vi "CTRE_PID.vi"(9 "Sensor Derivative":dbl, 10 "Servo Params":T1, 11 "Error":dbl) -> (2 "At Target":bool, 3 "Out":dbl)   [LabVIEW 2016]
uses:
  <vilib>/Rock Robotics/WPI/ThirdParty/CanMotor/CTRLib-LV-TalonSRX/Framework/ServoParams.ctl
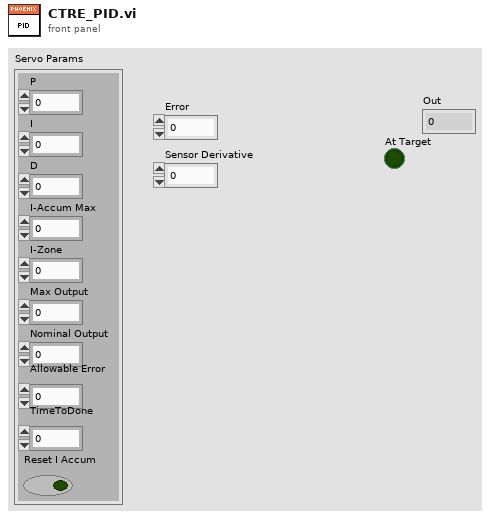
[diagram p1: front panel]
types:
  T1 = typedef "ServoParams.ctl" = cluster{"P":dbl, "I":dbl, "D":dbl, "I-Accum Max":dbl, "I-Zone":dbl, "Max Output":dbl, "Nominal Output":dbl, "Allowable Error":dbl, "TimeToDone":dbl, "Reset I Accum":bool}
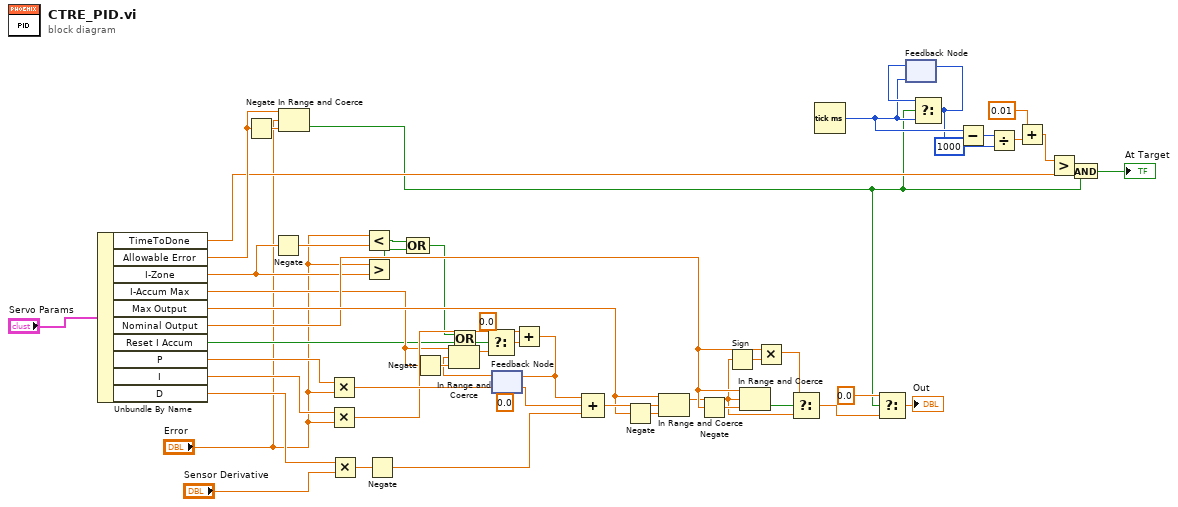
[diagram p0: block diagram]
diagram:
  n1 = Unbundle By Name("Servo Params") -> ("TimeToDone"=w10:dbl, "Allowable Error"=w17:dbl, "I-Zone"=w23:dbl, "I-Accum Max"=w29:dbl, "Max Output"=w38:dbl, "Nominal Output"=w35:dbl, "Reset I Accum"=w26:bool, "P"=w48:dbl, "I"=w47:dbl, "D"=w43:dbl)
  n2 = Negate(x=w17) -> (-x=w18:dbl)
  n3 = Negate(x=w23) -> (-x=w22:dbl)
  n4 = In Range and Coerce(upper limit=w17, x="Error", lower limit=w18) -> (In Range?=w6:bool)  [unwired: 1 out]
  n5 = Multiply(x=w48, y="Error") -> (x*y=w46:dbl)
  n6 = Multiply(x=w47, y="Error") -> (x*y=w45:dbl)
  n7 = Multiply(x=w43, y="Sensor Derivative") -> (x*y=w25:dbl)
  n8 = Less?(x="Error", y=w22) -> (x < y?=w20:bool)
  n9 = Greater?(x="Error", y=w23) -> (0:w21:bool)
  n10 = Negate(x=w25) -> (-x=w24:dbl)
  n11 = Compound Arithmetic op=OR(w20, w21) -> (w19:bool)
  n12 = Negate(x=w29) -> (-x=w31:dbl)
  n13 = Or(x=w19, y=w26) -> (x .or. y?=w27:bool)
  n14 = feedback #1(0.0) -> (w28:dbl)
  n15 = In Range and Coerce(upper limit=w29, x=w28, lower limit=w31) -> (coerced(x)=w30:dbl)  [unwired: 1 out]
  n16 = Select(t=0.0, s=w27, f=w30) -> (s? t:f=w42:dbl)
  n17 = Add(x=w45, y=w42) -> (x+y=w51:dbl)
  n18 = feedback-in #1(w51) -> ()
  n19 = Compound Arithmetic op=ADD(w51, w46, w24) -> (w40:dbl)
  n20 = Negate(x=w38) -> (-x=w39:dbl)
  n21 = In Range and Coerce(upper limit=w38, x=w40, lower limit=w39) -> (coerced(x)=w33:dbl)  [unwired: 1 out]
  n22 = Negate(x=w35) -> (-x=w37:dbl)
  n23 = Sign(1:w33) -> (0:w34:dbl)
  n24 = In Range and Coerce(upper limit=w35, x=w33, lower limit=w37) -> (In Range?=w36:bool)  [unwired: 1 out]
  n25 = Multiply(x=w35, y=w34) -> (x*y=w32:dbl)
  n26 = Select(t=w32, s=w36, f=w33) -> (s? t:f=w15:dbl)
  n27 = Tick Count (ms)() -> (millisecond timer value=w12:u32)
  n28 = Select(t=0.0, s=w6, f=w15) -> (s? t:f=→"Out":dbl)
  n29 = feedback #2(w12) -> (w13:u32)
  n30 = Select(t=w13, s=w6, f=w12) -> (s? t:f=w11:u32)
  n31 = feedback-in #2(w11) -> ()
  n32 = Subtract(x=w12, y=w11) -> (x-y=w5:u32)
  n33 = Divide(x=w5, y=u32 1000) -> (x/y=w3:dbl)
  n34 = Add(x=0.01, y=w3) -> (x+y=w1:dbl)
  n35 = Greater?(x=w1, y=w10) -> (0:w9:bool)
  n36 = And(x=w9, y=w6) -> (x .and. y?=→"At Target":bool)
